vi "Role Decisor Simple.vi"(0 "Receptor passe":enum16{"Auto", "2nd Striker", "Striker"}(ring), 6 "Pinned":T1={"Attc"="Auto", "Strk"="Auto", "Def"=[], "Strk 2"="Auto"}, 8 "Modo Teste ?":bool, 9 "Qtd Min p/ Stk":dbl=2.0, 11 "channel":T14) -> (2 "Output IA":T3, 3 "channel 2":T14)   [LabVIEW 2017]
uses:
  <extravilib>/ChannelInstances/Lossy Stream-t'AI Input.ctl'/)Channel.ctl
  Core/AI Input.ctl
  Core/AI Robot.ctl
  Intel/Functions Enum.ctl
  Intel/AttackerStates.ctl
  Path Planning/RRT/PathDests.ctl
  Path Planning/RRT/PathDest.ctl
  Core/AI Ball.ctl
  Core/Field Size.ctl
  Core/AI Judge.ctl
  Intel/Command Enum.ctl
  Util/Events/Events.ctl
  Select Personalitys.ctl
  Util/Select Auto None or Robot.ctl
  <extravilib>/ChannelInstances/Lossy Stream-t'AI Input.ctl'/Read With Abort.vi
  <extravilib>/ChannelInstances/Lossy Stream-t'AI Input.ctl'/Write With Abort.vi
  <extravilib>/ChannelInstances/Lossy Stream-t'AI Input.ctl'/EndpointRead.vi
  <extravilib>/ChannelInstances/Lossy Stream-t'AI Input.ctl'/Endpoint.vi
  <extravilib>/ChannelInstances/Lossy Stream-t'AI Input.ctl'/)Channel.vi
  <resource>/ChannelSupport/_ChannelSupport/WaitIfNeeded.vi
  <extravilib>/ChannelInstances/Lossy Stream-t'AI Input.ctl'.lvlib
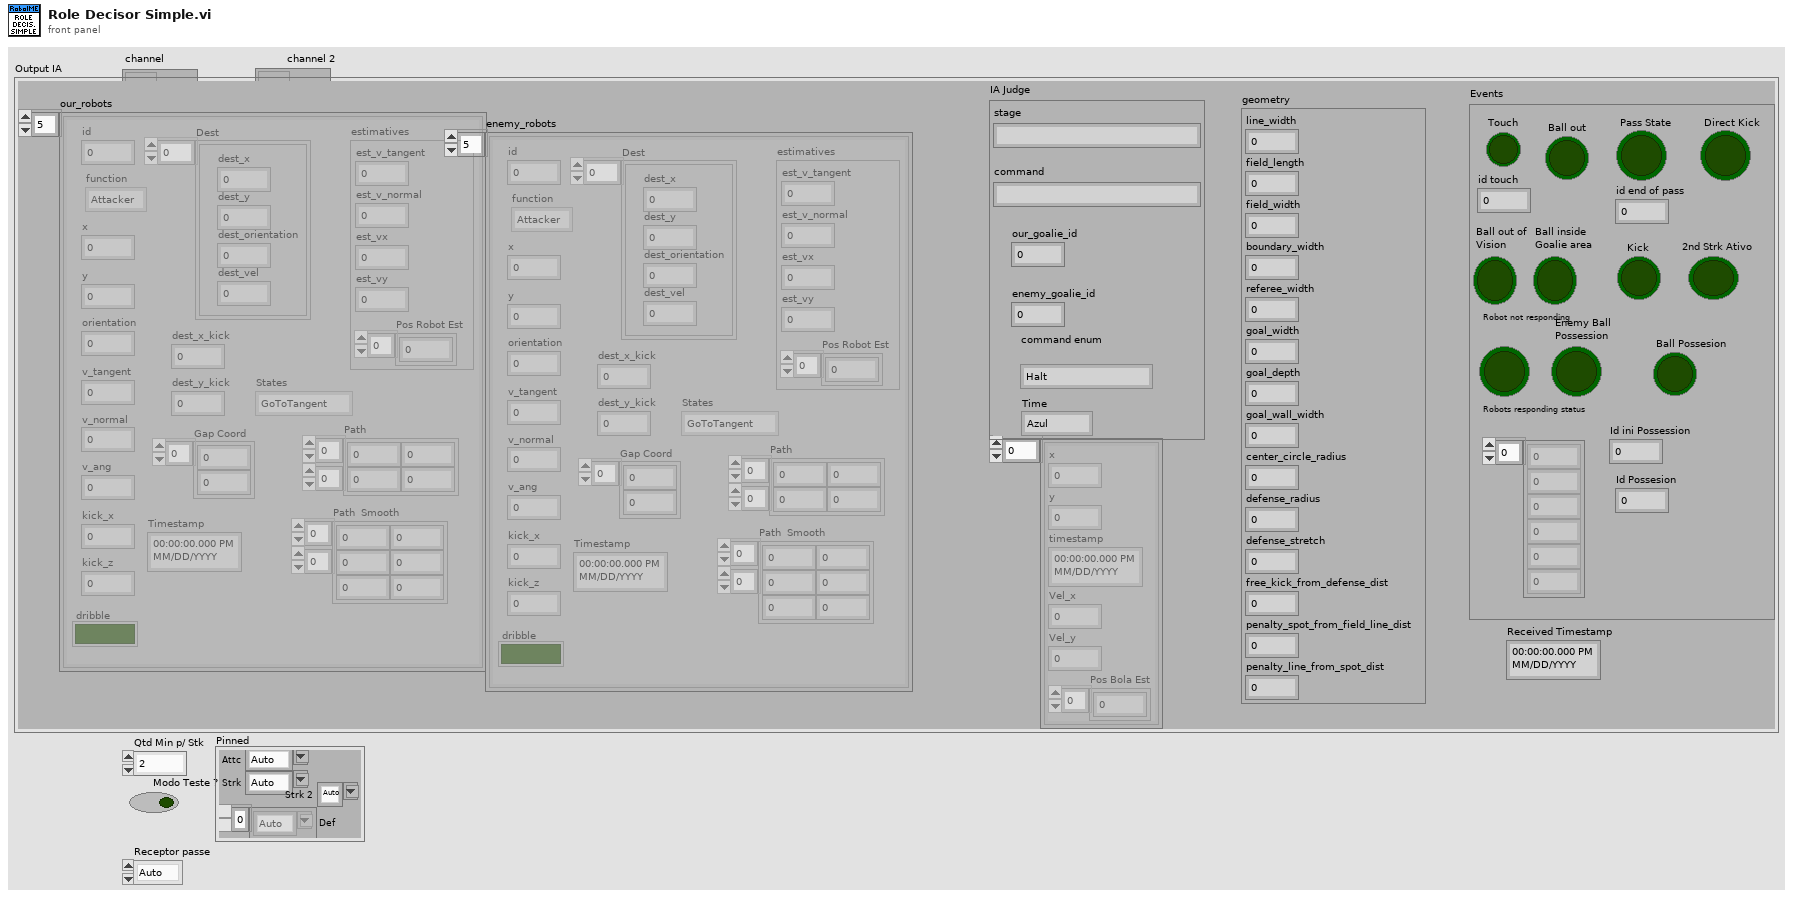
[diagram p1: front panel]
types:
  T1 = typedef "Select Personalitys.ctl" = cluster{"Attc":T2, "Strk":T2, "Def":T2[], "Strk 2":T2}
  T2 = typedef "Select Auto None or Robot.ctl" = string
  T3 = typedef "AI Input.ctl" = cluster{"our_robots":T4[], "enemy_robots":T4[], "balls":T9[], "geometry":T10, "IA Judge":T11, "Received Timestamp":timestamp, "Events":T13}
  T4 = typedef "AI Robot.ctl" = cluster{"id":u32, "function":T5, "x":dbl, "y":dbl, "orientation":dbl, "v_tangent":dbl, "v_normal":dbl, "v_ang":dbl, "kick_x":dbl, "kick_z":dbl, "dribble":bool, "Timestamp":timestamp, "estimatives":cluster{"est_v_tangent":dbl, "est_v_normal":dbl, "est_vx":dbl, "est_vy":dbl, "Pos Robot Est":dbl[]}, "dest_x_kick":dbl, "dest_y_kick":dbl, "Gap Coord":dbl[], "States":T6, "Path ":dbl[][], "Path  Smooth":dbl[][], "Dest":T7}
  T5 = typedef "Functions Enum.ctl" = enum16{"2nd Striker", "Attacker", "Goalie", "Defender", "Striker", "Goto 0", "Dummy", "Kicker", "ZigZag 0", "ZigZag 1", "ZigZag 2", "ZigZag 3", "ZigZag 4", "ZigZag 5", "ZigZag 6", "ZigZag 7", "ZigZag 8", ""}
  T6 = typedef "AttackerStates.ctl" = enum16{"Pass", "GoToTangent", "BallGetting", "GoToKick", ""}
  T7 = typedef "PathDests.ctl" = T8[]
  T8 = typedef "PathDest.ctl" = cluster{"dest_x":dbl, "dest_y":dbl, "dest_orientation":dbl, "dest_vel":dbl}
  T9 = typedef "AI Ball.ctl" = cluster{"x":dbl, "y":dbl, "timestamp":timestamp, "Vel_x":dbl, "Vel_y":dbl, "Pos Bola Est":dbl[]}
  T10 = typedef "Field Size.ctl" = cluster{"line_width":u32, "field_length":u32, "field_width":u32, "boundary_width":u32, "referee_width":u32, "goal_width":u32, "goal_depth":u32, "goal_wall_width":u32, "center_circle_radius":u32, "defense_radius":u32, "defense_stretch":u32, "free_kick_from_defense_dist":u32, "penalty_spot_from_field_line_dist":u32, "penalty_line_from_spot_dist":u32}
  T11 = typedef "AI Judge.ctl" = cluster{"stage":string, "command":string, "our_goalie_id":dbl, "enemy_goalie_id":dbl, "command enum":T12, "Time":enum16{"Azul", "Amarelo"}}
  T12 = typedef "Command Enum.ctl" = enum16{"Halt", "Stop", "Force Start", "PKA Normal Start", "Prepare Kickoff Ally", "PKE Normal Start", "Prepare Kickoff Enemy", "Prepare Penalty Ally", "PPA Normal Start", "Prepare Penalty Enemy", "PPE Normal Start", "Direct Free Enemy", "Direct Free Ally", "Indirect Free Enemy", "Indirect Free Ally", "Timeout Enemy", "Timeout Ally", "Goal Enemy", "Goal Ally", "Ball Placement Enemy", "Ball Placement Ally", "Normal Half Time", "Extra Time Break", "Extra Half Time", "None", "Post Game"}
  T13 = typedef "Events.ctl" = cluster{"Touch":bool, "Ball out":bool, "id touch":dbl, "Ball out of \nVision":bool, "Ball inside \nGoalie area":bool, "Robot not responding":bool, "Robots responding status":dbl[], "Enemy Ball \nPossession":bool, "Pass State":bool, "id end of pass":dbl, "Kick":bool, "Id ini Possession":dbl, "Ball Possesion":bool, "Id Possesion":dbl, "Direct Kick":bool, "2nd Strk Ativo":bool}
  T14 = typedef "Lossy Stream-t'AI Input.ctl'.lvlib/)Channel.ctl" = refnum<queue>
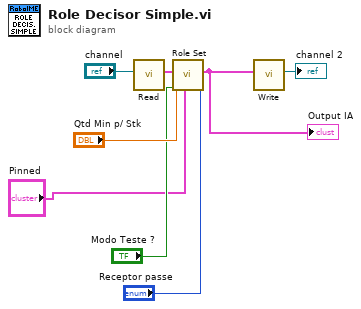
[diagram p0: block diagram]
diagram:
  n1 = call <extravilib>:"Read.vi"("channel"="channel") -> ("element"=w8:T3)  [unwired: 5 in, 5 out]
  n2 = call "Role Set.vi"("Receptor passe"="Receptor passe", "Pinned"="Pinned", "Modo Teste ?"="Modo Teste ?", "Qtd Min p/ Stk"="Qtd Min p/ Stk", "Output IA Input"=w8) -> ("Output IA"=w5:T3)  [unwired: 6 in]
  "Output IA" <- w5
  n3 = call <extravilib>:"Write.vi"("element"=w5) -> ("channel"=→"channel 2":T14)  [unwired: 8 in, 2 out]
